vi "List - Up Index.vi"(8 "Error In":errorcluster, 10 "Index":i32, 11 "List In":string[](array[string])) -> (0 "Error Out":errorcluster, 3 "List Out":cluster{"Name":string, "Selected":bool}[](array[cluster]))   [LabVIEW 2020]
doc: "This VI use to set the value as False."
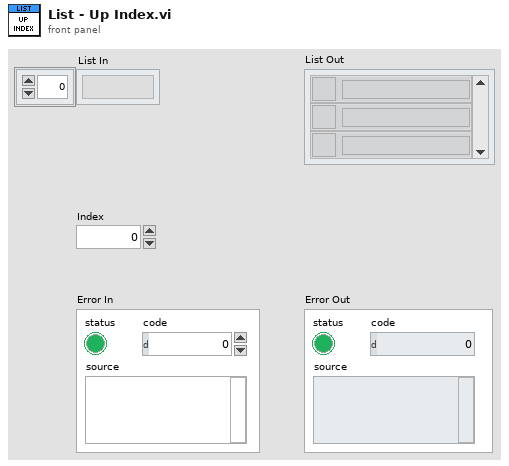
[diagram p1: front panel]
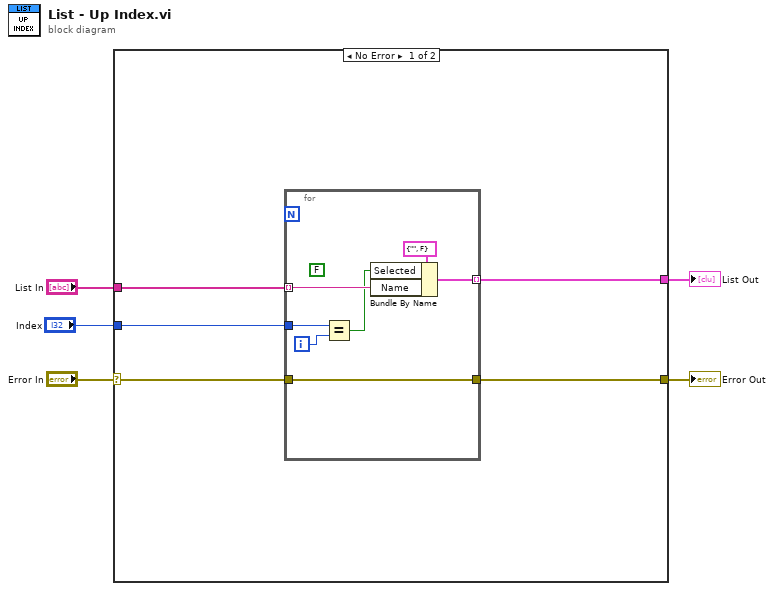
[diagram p0: block diagram]
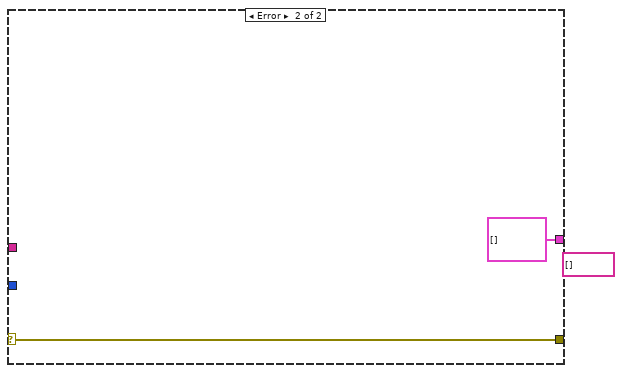
[diagram p2: hidden frame]
diagram:
  n1 = case shown="No Error" "Error In" {
    selector: "Error In" -> [w10 w19]
    tunnel: [w9 w19] -> w4
    tunnel: "List In" -> [w8 _]
    tunnel: [w7 cluster{"Name":string, "Selected":bool}[] []] -> w2
    tunnel: "Index" -> [w6 _]
    frame No Error {
      n2 = for {
        tunnel: w8 -> [w16] mode=indexing
        tunnel: [w17] -> w9
        tunnel: w10 -> [w17]
        tunnel: [w14] -> w7 mode=indexing
        tunnel: w6 -> [w13]
        i -> [w12]
        (unwired) FALSE ("Selected")
        n3 = Equal?(x=w13, y=w12) -> (x = y?=w11:bool)
        n4 = Bundle By Name(cluster=cluster{"Name":string, "Selected":bool} {"Name"="", "Selected"=FALSE} ("File List"), "Selected"=w11, "Name"=w16) -> (w14:cluster{"Name":string, "Selected":bool})
      }
    }
    frame Error {
      (unwired) string[] []
      (unwired) string[] []
    }
  }
  "Error Out" <- w4
  "List Out" <- w2
